vi "Combine TDMS Files.vi"   [LabVIEW 2015]
doc: "This VI will combine several <B>TDMS Files</B> into a single <B>Combined TDMS Path</B>. If the combine operation performed a successful copy then the <b>Success?</b> will be <b>TRUE</b>. Note that this simply means the merge was successful, it does not mean the output is valid.\n\n-----\nBrian Hoover (Hooovahh)"
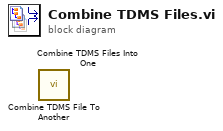
[diagram p0: block diagram]
diagram:
  n1 = call "Combine TDMS File To Another.vi"() -> ()  [unwired: 10 in, 2 out]
  n2 = call "Combine TDMS Files Into One.vi"() -> ()  [unwired: 10 in, 2 out]
